vi "Read Rate (Hz).vi"(8 "error in (no error)":errorcluster, 11 "Change Blue Laser Rate MSG in":refnum<class "Change Blue Laser Rate MSG.lvclass">) -> (0 "error out":errorcluster, 2 "Rate (Hz)":i32, 3 "Change Blue Laser Rate MSG out":refnum<class "Change Blue Laser Rate MSG.lvclass">)   [LabVIEW 2014, in "eCRDS Library.lvlib" / "Change Blue Laser Rate MSG.lvclass"]
uses:
  Change Blue Laser Rate MSG.lvclass
  Change Blue Laser Rate MSG.lvclass/Change Blue Laser Rate MSG.ctl
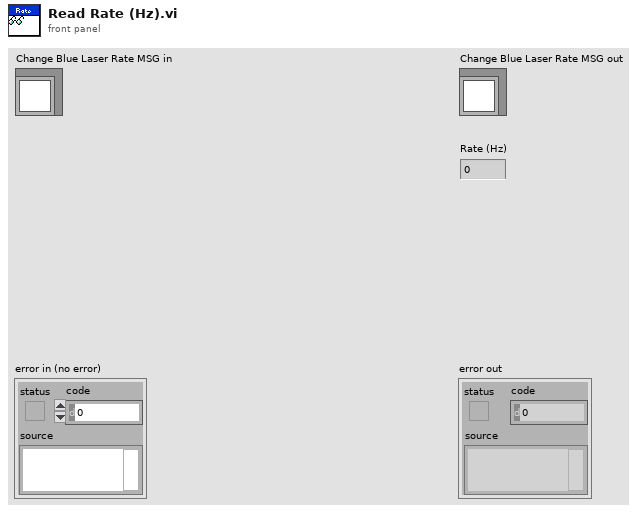
[diagram p1: front panel]
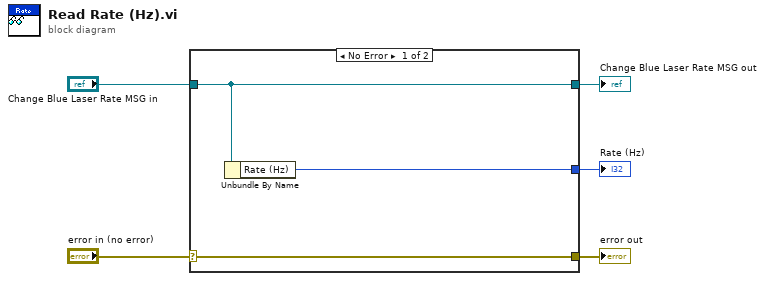
[diagram p0: block diagram]
diagram:
  n1 = case shown="No Error" "error in (no error)" {
    selector: "error in (no error)" -> [w8 w9]
    tunnel: [w8 w9] -> w4
    tunnel: [w7 w10] -> w2
    tunnel: "Change Blue Laser Rate MSG in" -> [w7 w10]
    tunnel: [w6 _] -> w1
    frame No Error {
      n2 = Unbundle By Name(w7) -> ("Rate (Hz)"=w6:i32)
    }
    frame Error {
    }
  }
  "error out" <- w4
  "Change Blue Laser Rate MSG out" <- w2
  "Rate (Hz)" <- w1
